vi "csv_control _03.vi"() -> ()   [LabVIEW 2024]
panel:
  in  "SN 2":string
  in  "Test_ID 2":string
  in  "Test_Value 2":dbl
  out "添加的数组":string[](array[string])
  in  "Test_Value":dbl
  in  "Test_ID":string
  in  "SN":string
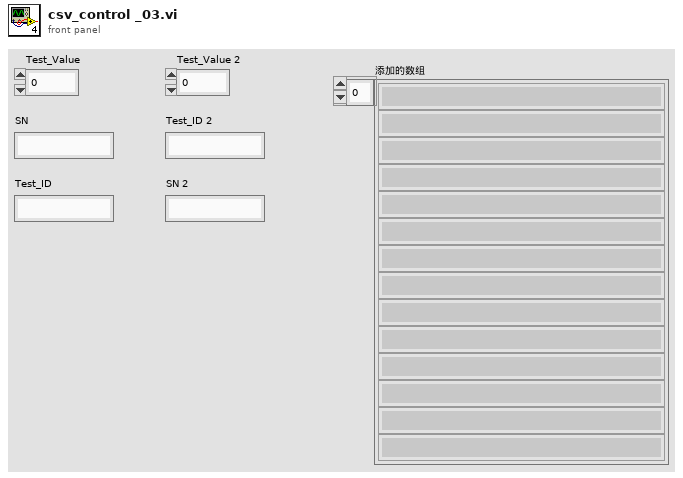
[diagram p1: front panel]
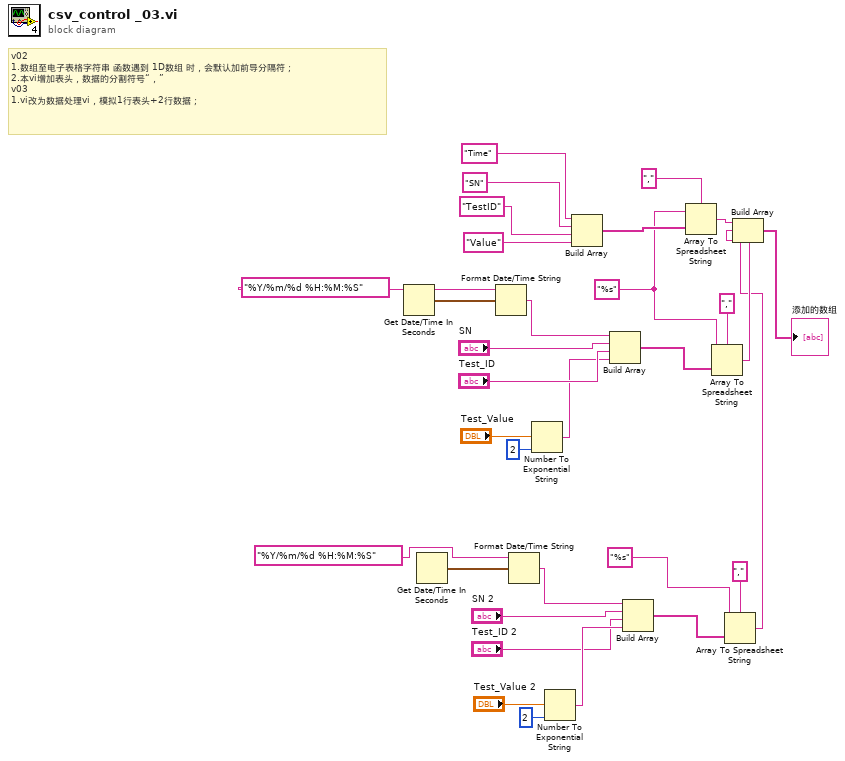
[diagram p0: block diagram]
diagram:
  w17 = "%s" ("格式字符串")
  # "v02\n1.数组至电子表格字符串 函数遇到 1D数组 时，会默认加前导分隔符；\n2.本vi增加表头，数据的分割符号“，”\nv03\n1.vi改为数据处理vi，模拟1行表头+2行数据；"
  n1 = Get Date/Time In Seconds() -> (seconds since 1Jan1904=w28:timestamp)
  n2 = Get Date/Time In Seconds() -> (seconds since 1Jan1904=w7:timestamp)
  n3 = Format Date/Time String(time format string (%c)="%Y/%m/%d %H:%M:%S" ("时间格式字符串(%c)"), seconds (now)=w28) -> (date/time string=w24:string)  [unwired: 1 in]
  n4 = Format Date/Time String(time format string (%c)="%Y/%m/%d %H:%M:%S" ("时间格式字符串(%c)"), seconds (now)=w7) -> (date/time string=w10:string)  [unwired: 1 in]
  n5 = Number To Exponential String(number="Test_Value", precision (6)=i16 2 ("精度(6)")) -> (E-format string=w29:string)  [unwired: 2 in]
  n6 = Number To Exponential String(number="Test_Value 2", precision (6)=i16 2 ("精度(6)")) -> (E-format string=w6:string)  [unwired: 2 in]
  n7 = Build Array("Time" ("元素"), "SN" ("元素"), "TestID" ("元素"), "Value" ("元素")) -> (w18:string[])
  n8 = Build Array(w24, "SN", "Test_ID", w29) -> (w26:string[])
  n9 = Build Array(w10, "SN 2", "Test_ID 2", w6) -> (w8:string[])
  n10 = Array To Spreadsheet String(delimiter (Tab)="," ("分隔符(Tab)"), array=w18, 3:w17) -> (spreadsheet string=w15:string)
  n11 = Array To Spreadsheet String(delimiter (Tab)="," ("分隔符(Tab)"), array=w26, 3:w17) -> (spreadsheet string=w14:string)
  n12 = Array To Spreadsheet String(delimiter (Tab)="," ("分隔符(Tab)"), array=w8, 3:"%s" ("格式字符串")) -> (spreadsheet string=w1:string)
  n13 = Build Array(w15, w14, w1) -> (→"添加的数组":string[])
